vi "Spectrophotometer.vi"() -> ()   [LabVIEW 2015]
uses:
  lamp 3.ctl
  measurement mode.ctl
  standard cluster 2.ctl
  settings.ctl
  sample cluster.ctl
panel:
  in  "Export":bool
  in  "Quick Measure":bool
  in  "Quit":bool
  in  "Mixture Analysis":bool
  in  "Turn Lamp on/off":bool
  in  "Measure reference":bool
  in  "Continuous Sampling":bool
  in  "Print":bool
  in  "Run Pump":bool
  in  "Load Unknowns":bool
  in  "Load Standards":bool
  in  "Measure Unknowns":bool
  in  "Measure Standards":bool
  out "mse":dbl format="%.2e"
  out "Sample cluster":T1={"General description"="", "Sample setup"={"integration time"=0.5, "rinse time"=10.0, "sample time"=10.0, "sample type"=0}, "Absorbance"=[], "Analyst"="", "Sample descriptions"=[], "good data"=[]} {"Absorbance" format="%.2e"; "Sample setup"."sample type" items=["Sample Cuvet", "Sipper Cell", "No Dialog"]; "Sample setup"."sample time" min=0.0 max=100.0 step=1.0 format="%.1f"; "Sample setup"."rinse time" min=0.0 max=100.0 step=1.0 format="%.1f"; "Sample setup"."integration time" format="%.1f"}
  out "standard cluster":T3={"Description"="", "Setup"={"integration time"=0.5, "rinse time"=10.0, "sample time"=10.0, "sample type"=0}, "Concentrations"=[], "Absorbance"=[], "Analyst"="", "Concentration units"="", "Good"=[]} {"Absorbance" format="%.2e"; "Concentrations" format="%.2p"; "Setup"."sample type" items=["Sample Cuvet", "Sipper Cell", "No Dialog"]; "Setup"."sample time" min=0.0 max=100.0 step=1.0 format="%.1f"; "Setup"."rinse time" min=0.0 max=100.0 step=1.0 format="%.1f"; "Setup"."integration time" format="%.1f"}
  out "Max Abs":dbl[](array[numeric])=[2.5701224514044116, 2.7143632947038925, 2.7377490738915573, 2.781755374652469, 2.7830312576242777, 2.8032522114304568, 2.7921527618220714, 2.7673636837963227, 2.7721309273843646, 2.765787727286867, 2.807007059774088, 2.7902851640332416, 2.832726005678466, 2.8510992821765293, 2.8064913329195997, 2.8579954955609237, 2.826035908916132, 2.7882815275987913, 2.827020146123574, 2.862584527170188, 2.8696657972102946, 2.870029150013057, 2.850339854583479, 2.8344461374598717, 2.810178732066239, 2.898747115100364, 2.8854629958743176, 2.8929623242217075, 2.897616096354254, 2.8235133530369914, 2.842072279560508, 2.8740060946591246, 2.8952788625213643, 2.9197995727392203, 2.7718078789991054, 2.7746483290640764, 2.9113813592906737, 2.8881008306142317, 2.8491859254377956, 2.913029295578773, 2.8686091762476096, 2.9204468386734073, 2.88930170250631, 2.884183410137873, 2.874273027848105, 2.8890999188452047, 2.897462138013063, 2.926856708949692, 2.868338737959064, 2.905860615093137, 2.835906080237521, 2.8753391229545393, 2.9027206797044833, 2.7781657266251045, 2.7936088088519138, 2.8090207204836726, 2.809411557915602, 2.8104475951231165, 2.798402011467731, 2.7894114735514233, 2.9238654751855013, 2.9081953926712476, 2.8844894948295754, 2.868914686447694, 2.8460648194194156, 2.933922376656966, 2.9145335490140183, 2.9086029593887113, 2.8939059482930922, 2.893051223353465, 2.884444162559301, 2.889872914270699, 2.885485609489626, 2.896151283804924, 2.8967245808281366, 2.910314846434508, 2.9140468259476626, 2.929408706900379, 2.9352653639533064, 2.9521237832016056, 2.9551680174761126, 2.870181433343178, 2.8722378774668362, 2.8840019247687874, 2.8835592361928204, 2.8905663182570516, 2.8863666233051126, 2.9627101964477114, 2.9386998099696515, 2.91425851170049, 2.9100478084869774, 2.905612412895181, 2.892739996745825, 2.899097900707322, 2.8947147215259488, 2.9053640687668922, 2.9628994480115844, 2.9634572601167077, 2.9468843793177224, 2.964504765269017, 2.9391297105036522, 2.9489506102455483, 2.958143240475256, 2.943237226575327, 2.9568308966253545, 2.957760484109844, 2.925569909543376, 2.9320981608102477, 2.9437318785364797, 2.983147984219146, 2.918565007974718, 2.9265893685399558, 2.940964493492799, 2.9274114291335085, 2.9227877179721355, 2.9445813642269263, 2.9180093558683367, 2.9153470623241917, 2.958516103423041, 2.988112840268352, 2.9362120443202486, 2.988665956710447, 2.915821787620399, 2.9916424442139777, 2.914713286973624, 2.924134497101746, 2.980367026184775, 2.9828770130682005, 2.974695871909683, 2.9668266733534754, 2.9595183769729982, 2.944650435338738, 2.920332071539589, 2.932453470068308, 2.953682391064328, 2.95193947855959, 2.983120894710853, 2.9466487339066765, 2.9510362257417495, 2.970625776688294, 2.962037686565013, 2.963362766103736, 2.9864582127373063, 2.9954070203944414, 2.971758130277843, 2.9846263122003296, 2.9966167306916187, 3.0002344557228784, 2.899535984652174, 2.989627770745151, 2.942959975186675, 2.9796849238270258, 2.9614780469852766, 2.9584683183669434, 2.975275526294007, 2.9971853565284476, 2.992270670437009, 2.9737834204390037, 2.977970397281164, 2.996152530275524, 2.967416919318192, 2.970607188895619, 2.9724250217818824, 2.995977231283496, 2.991305836741952, 2.993991419687998, 2.9771014330008883, 2.989405318001516, 2.9697978489463743, 2.988674872173253, 2.977257059654726, 2.985336641735613, 2.9766800457593336, 2.993241746483962, 2.9943787503552803, 2.9852288183853912, 2.9900367863183996, 2.9793115878060052, 2.993718320050437, 2.9663388811545617, 2.9916158794231995, 2.9982680591088706, 2.9787737843301225, 2.9764416893788446, 2.993938575094718, 2.9830305841443057, 2.9811024954238863, 2.9745853737795214, 2.9796849238270258, 2.9502869470332103, 2.9790837862828363, 2.940556326635444, 3.007577098304339, 2.9971328991685695, 2.9268669879873825, 2.8809621413005586, 2.9915007465494234, 2.986386518883215, 2.893595333819883, 2.8948696567452523, 2.920811805185074, 2.9529860651970554, 2.8761023213777936, 2.9825425823029432, 2.961231197044663, 2.864261824184963, 3.002667047908652, 2.8475849968782785, 2.9785183223473086, 2.966948535845015, 2.976954909894943, 2.9797122285003805, 2.9877466823844996, 2.9517065608430424, 2.973561931079017, 2.9507930951262478, 2.9857945925606715, 2.959251330111692, 2.9697233511042374, 2.9754226169943916, 2.987916403689377, 2.9795847920016643, 2.9802125101844354, 2.9975349104293665, 2.969238803388194, 3.002563443006112, 2.902253164413887, 2.9254668006915376, 2.881567238929719, 2.9765425484286254, 2.982099290774663, 2.9982506175634103, 2.844588996837636, 2.9800306562438332, 2.9985378777712164, 3.0004340774793183, 2.9470610295060045, 2.8992074631292315, 2.8633466564264207, 2.827808515509827, 2.83905045598111, 2.989965680840462, 2.87559367147926, 2.873831919363592, 2.920144205331227, 2.9868165045855366, 2.9401577450345013, 3.0014394694805917, 2.9767167043633824, 3.001949941084268, 2.9683054586308106, 2.995775549929434, 2.988273495044722, 2.9498484576324793, 2.982596831816711, 2.9495461294045358, 2.9017306917292185, 2.9264144800205227, 2.8723544290433782, 2.985857410884626, 2.941163460158473, 2.938989289805111, 2.981066205174902, 2.990817735602789, 2.8994374542861774, 2.9779064276371185, 2.9417796781737486, 2.9370964319634765, 2.981963498779465, 3.0066286048286996, 2.9856150615513544, 3.0025202670010356, 2.9894854141161935, 2.9764141782996054, 2.978271841610635, 3.004699604225055, 2.984787811891183, 2.963277703909644, 2.9347407805432075, 2.985480364573659, 2.9774400784660493, 2.983193129645013, 2.9729795213258945, 2.9958106316760427, 2.9554087118535692, 2.9892183696006756, 2.9759829437125465, 2.9923060364371836, 2.9796212062457554, 2.9712846644554203, 2.9653334280184214, 2.968277427274059, 2.9958194016699227, 2.928825836692016, 2.913866811896239, 2.9962401532444884, 2.989075878689533, 3.002407989295258, 2.958085848521085, 2.9812381033887854, 3.0012922730241685, 2.9299703849090117, 2.972072715743075, 3.010850957373923, 2.865743391885155, 2.895024536710891, 2.8531260748344462, 2.8453461374114086, 2.8730996193611147, 2.976056375590289, 2.8718997009048017, 2.809855876532671, 2.7851019486186024, 2.8378030074943434, 2.751048034820188, 2.7677938472611476] format="%.2f"
  out "Sample absorbance":dbl[](array[numeric])=[0.07717] format="%.4f"
  out "concentration":dbl=0.0001 format="%.1e"
  in  "measurement mode":T4 {"gain" max=15}
  out "lamp":T5
  out "max. conc.":dbl format="%.2p"
  out "reference":bool=TRUE
  out "calibration graph":cluster{dbl[], dbl[]}[](graph)
  out "Sample concentration":dbl[](array[numeric])=[0.00011953621702929448] format="%.2e"
  out "Sample description":string[](array[string])
  out "Samples graph":cluster{sgl, sgl, dbl[][]}(graph)
  out "r":dbl format="%.4f"
  out "intercept":dbl format="%.2e"
  out "slope":dbl format="%.3e"
  in  "GPIB":string="18"
  out "Standards graph":cluster{sgl, sgl, dbl[][]}(graph)
  # "nm"
  # "absorbance"
  # "Calibration graph"
  # "Description"
  # "Absorbance"
  # "Concentration"
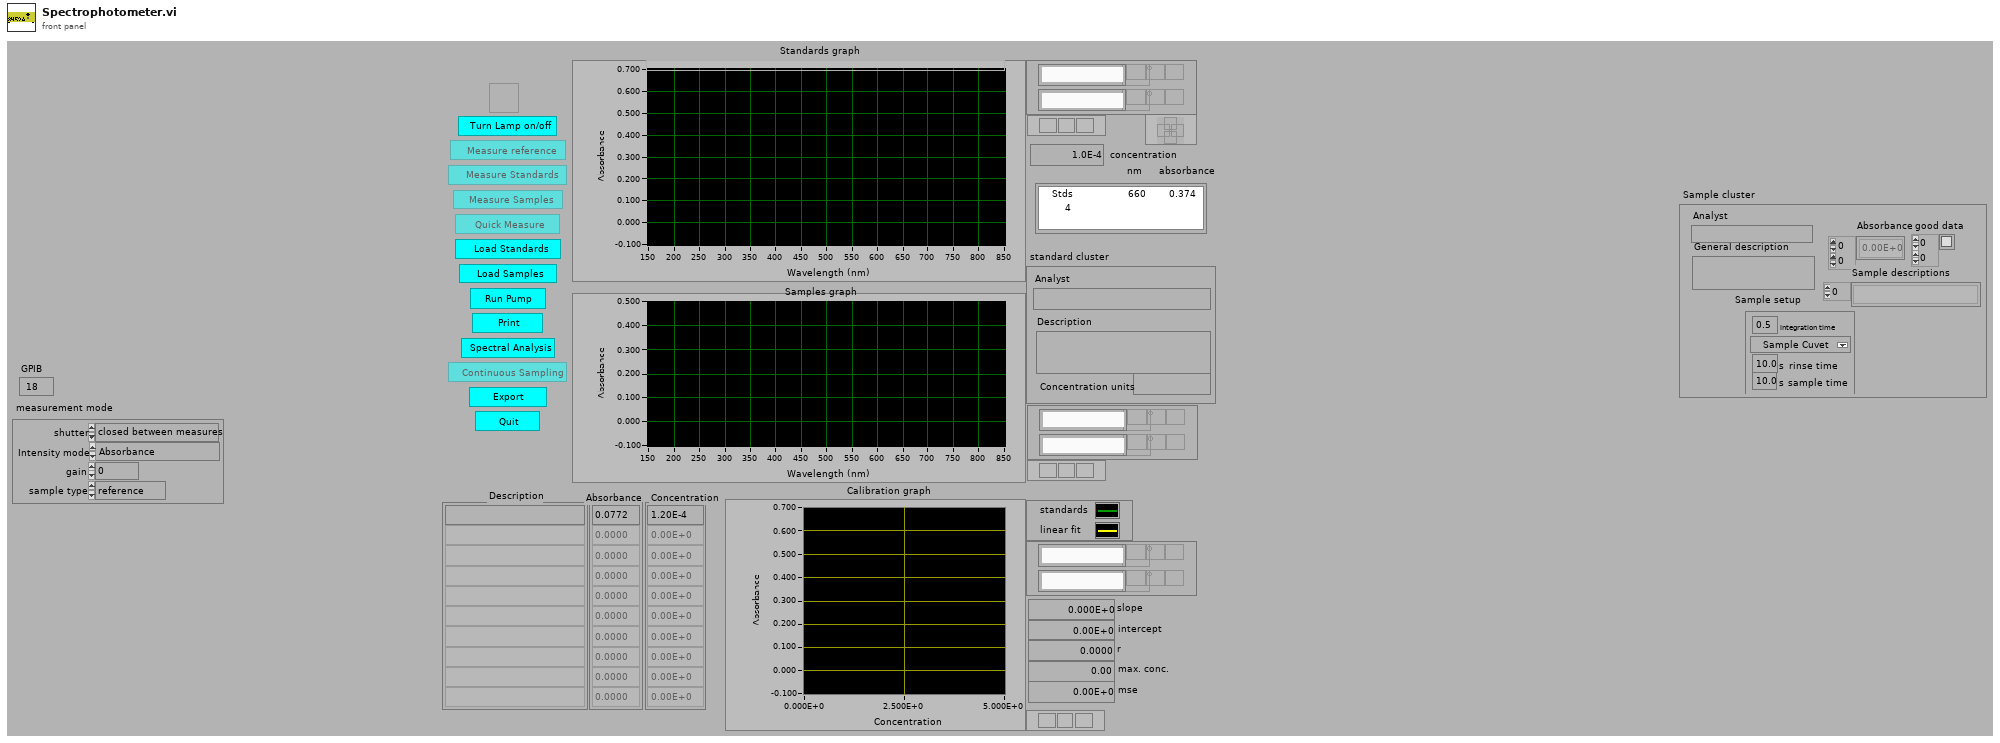
[diagram p1: front panel]
types:
  T1 = typedef "sample cluster.ctl" = cluster{"General description":string, "Sample setup":T2, "Absorbance":dbl[][], "Analyst":string, "Sample descriptions":string[], "good data":bool[][]}
  T2 = typedef "settings.ctl" = cluster{"integration time":sgl, "rinse time":dbl[unit], "sample time":dbl[unit], "sample type":u16}
  T3 = typedef "standard cluster 2.ctl" = cluster{"Description":string, "Setup":T2, "Concentrations":dbl[], "Absorbance":dbl[][], "Analyst":string, "Concentration units":string, "Good":bool[][]}
  T4 = typedef "measurement mode.ctl" = cluster{"shutter":enum16{"closed between measures", "open between measures"}, "Intensity mode":enum16{"Absorbance", "Intensity at current gain", "Intensity at fixed gain", "dark current at current gain", "dark current at fixed gain"}, "gain":u8, "sample type":enum16{"reference", "standard", "unknown", "Diagnostic"}}
  T5 = typedef "lamp 3.ctl" = bool
  T6 = enum16{"reference", "standard", "unknown", "Diagnostic"}
  T7 = typedef "lamp2.ctl" = bool
  T8 = typedef "standard cluster.ctl" = cluster{"Description":string, "Setup":T2, "Concentrations":dbl[], "Absorbance":dbl[][], "Analyst":string, "Concentration units":string, "Good":bool[][]}
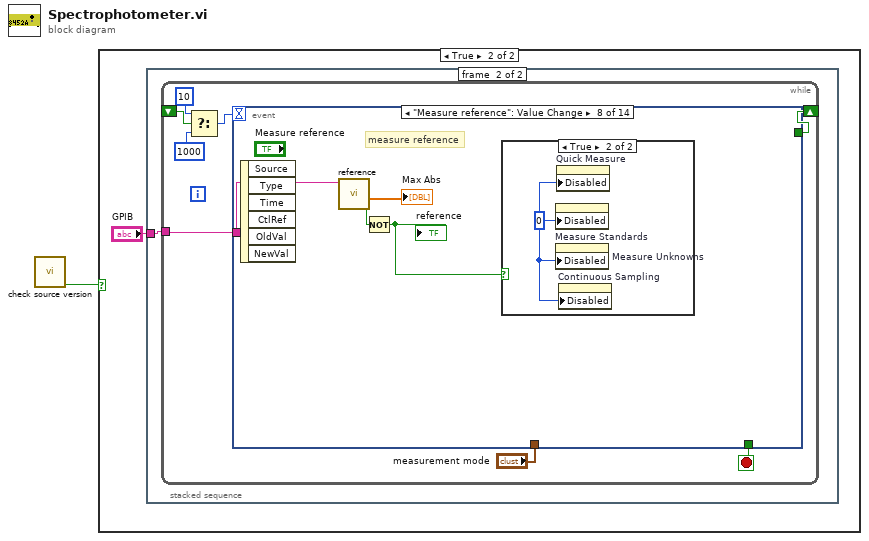
[diagram p0: block diagram]
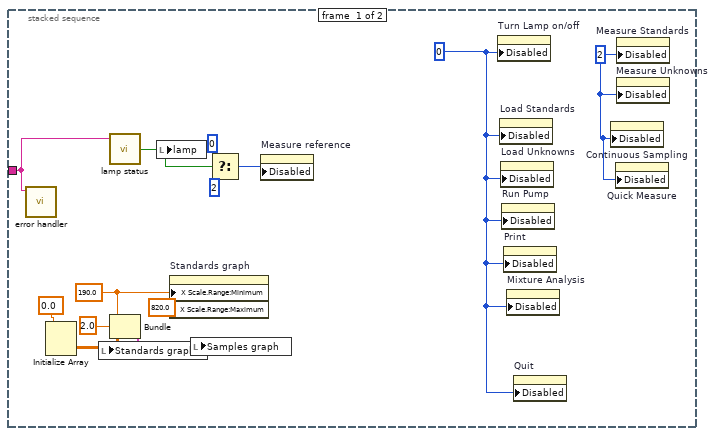
[diagram p3: hidden frame]
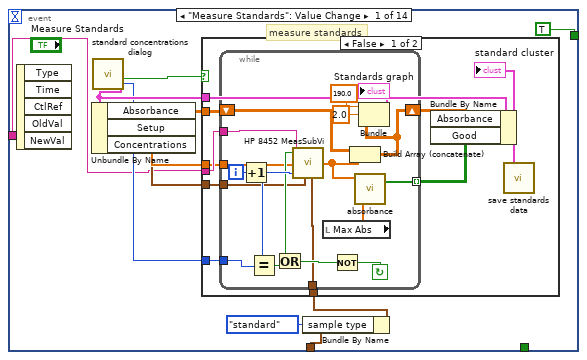
[diagram p4: hidden frame]
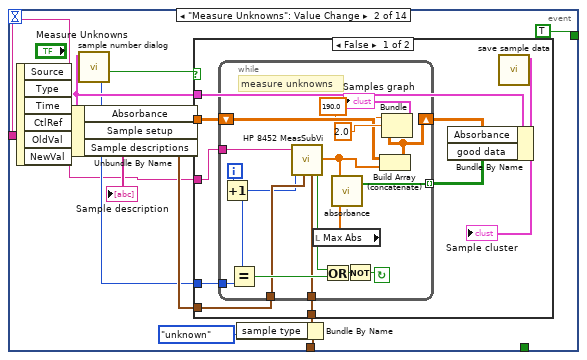
[diagram p6: hidden frame]
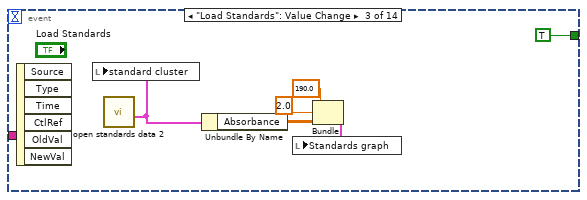
[diagram p8: hidden frame]
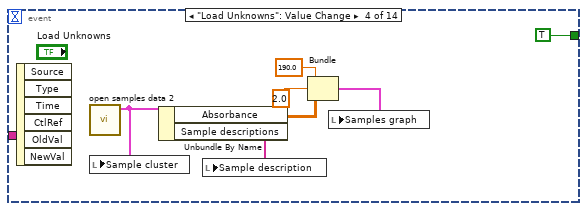
[diagram p9: hidden frame]
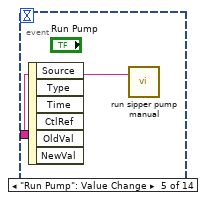
[diagram p10: hidden frame]
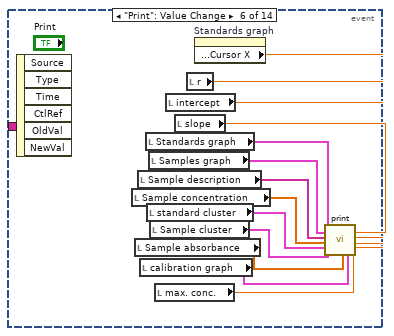
[diagram p11: hidden frame]
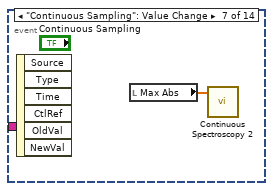
[diagram p12: hidden frame]
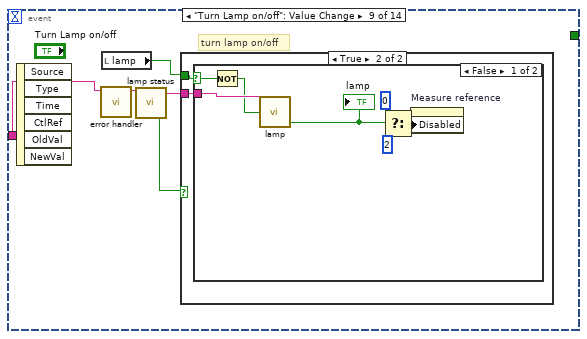
[diagram p14: hidden frame]
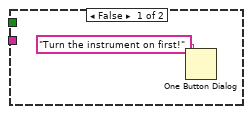
[diagram p15: hidden frame]
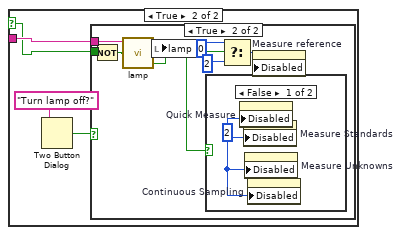
[diagram p16: hidden frame]
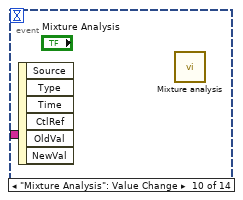
[diagram p19: hidden frame]
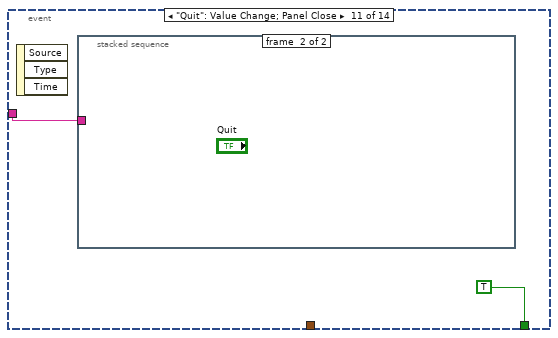
[diagram p20: hidden frame]
diagram:
  n1 = call "check source version.vi"() -> ("continue running?"=w1:bool)  [unwired: 2 in, 3 out]
  n2 = case shown="True" w1 {
    frame False {
    }
    frame True {
      n3 = stacked-sequence {
        tunnel: "GPIB" -> [w10 w16]
        frame #0 {
          w3 = 2
          w11 = 0
          w13 = sgl 190.0
          n4 = call "error handler.vi"("GPIB in"=w10) -> ()  [unwired: 4 in, 3 out]
          n5 = Initialize Array(0.0) -> (w5:dbl[][])  [unwired: 2 in]
          n6 = call "lamp status.vi"("GPIB in"=w10) -> ("lamp"=w6:T7)  [unwired: 2 in, 2 out]
          n7 = Bundle(w13, sgl 2.0, w5) -> (w4:cluster{sgl, sgl, dbl[][]})  [unwired: 1 in]
          n8 = local write "Standards graph"(w4) -> ()
          n9 = local write "lamp"(w6) -> ()
          n10 = property on="Standards graph" class="WFGraph (strict)"("X Scale.Range:Minimum"=w13, "X Scale.Range:Maximum"=sgl 820.0) -> ()  [unwired: 2 in, 2 out]
          n11 = local write "Samples graph"(w4) -> ()
          n12 = Select(t=0, s=w6, f=2) -> (s? t:f=w7:i32)
          n13 = property on="Measure reference" class="Bool"("Disabled"=w7) -> ()  [unwired: 2 in, 2 out]
          n14 = property on="Turn Lamp on/off" class="Bool"("Disabled"=w11) -> ()  [unwired: 2 in, 2 out]
          n15 = property on="Load Standards" class="Bool"("Disabled"=w11) -> ()  [unwired: 2 in, 2 out]
          n16 = property on="Load Unknowns" class="Bool"("Disabled"=w11) -> ()  [unwired: 2 in, 2 out]
          n17 = property on="Run Pump" class="Bool"("Disabled"=w11) -> ()  [unwired: 2 in, 2 out]
          n18 = property on="Print" class="Bool"("Disabled"=w11) -> ()  [unwired: 2 in, 2 out]
          n19 = property on="Mixture Analysis" class="Bool"("Disabled"=w11) -> ()  [unwired: 2 in, 2 out]
          n20 = property on="Quit" class="Bool"("Disabled"=w11) -> ()  [unwired: 2 in, 2 out]
          n21 = property on="Continuous Sampling" class="Bool"("Disabled"=w3) -> ()  [unwired: 2 in, 2 out]
          n22 = property on="Quick Measure" class="Bool"("Disabled"=w3) -> ()  [unwired: 2 in, 2 out]
          n23 = property on="Measure Standards" class="Bool"("Disabled"=w3) -> ()  [unwired: 2 in, 2 out]
          n24 = property on="Measure Unknowns" class="Bool"("Disabled"=w3) -> ()  [unwired: 2 in, 2 out]
        }
        frame #1 {
          n25 = while {
            tunnel: w16 -> [w22]
            shift-right: [w19] -> _
            shift-left: _ -> [w18]
            stop <- w23 stop-if-true
            n26 = Select(t=10, s=w18, f=1000) -> (s? t:f=w17:i32)
            n27 = event shown="[7] \"Measure reference\": Value Change" {
              selector: _ -> [_ _ _ _ _ _ _ _ _ _ _ _ _ _]
              dyn-events: _ -> [_ _ _ _ _ _ _ _ _ _ _ _ _ _]
              timeout: w17 -> [_ _ _ _ _ _ _ _ _ _ _ _ _ _]
              tunnel: w22 -> [w28 w67 _ _ w116 _ _ w131 w136 _ w164 w176 w199 _]
              tunnel: "measurement mode" -> [w27 w68 _ _ _ _ _ _ _ _ _ _ w198 _]
              tunnel: [_ _ _ _ _ _ _ _ _ _ TRUE ("Quit") _ _ _] -> w23
              tunnel: [TRUE TRUE TRUE TRUE _ _ _ _ _ _ _ FALSE TRUE _] -> w19
              event "Measure Standards": Value Change {
                n28 = event-data() -> ()  [unwired: 1 in, 5 out]
                n29 = call "standard concentrations dialog"() -> ("canceled"=w31:bool, "number"=w29:i8, "standard cluster"=w34:T8)  [unwired: 9 in]
                n30 = Unbundle By Name(w34) -> ("Absorbance"=w33:dbl[][], "Setup"=w32:T2, "Concentrations"=w35:dbl[])
                n31 = Bundle By Name(cluster=w27, "sample type"=T6."standard") -> (w30:T4)
                n32 = case shown="False" w31 {
                  tunnel: w28 -> [w45 _]
                  tunnel: w30 -> [w44 _]
                  tunnel: w29 -> [w43 _]
                  tunnel: w33 -> [w42 _]
                  tunnel: w32 -> [w41 _]
                  tunnel: w34 -> [w40 _]
                  tunnel: w35 -> [w37 _]
                  frame False {
                    # "measure standards"
                    n33 = while {
                      tunnel: w37 -> [w47]
                      tunnel: [w48] -> w38 mode=indexing
                      tunnel: w41 -> [w50]
                      tunnel: w44 -> [w52]
                      tunnel: w43 -> [w56]
                      tunnel: w45 -> [w55]
                      shift-left: w42 -> [w64]
                      shift-right: [w63] -> w39
                      i -> [w61]
                      stop <- w57 continue-if-true
                      n34 = Increment(x=w61) -> (x+1=w54:i32)
                      n35 = Equal?(x=w54, y=w56) -> (x = y?=w59:bool)
                      n36 = call "HP 8452 MeasSubVi.vi"("GPIB in"=w55, "Standard"=w47, "sample number"=w54, "setup"=w50, "measurement mode"=w52) -> ("canceled"=w53:bool, "measurement"=w49:dbl[])  [unwired: 2 in, 1 out]
                      n37 = Or(x=w53, y=w59) -> (x .or. y?=w58:bool)
                      n38 = local read "Max Abs"() -> (w51:dbl[])
                      n39 = Not(x=w58) -> (.not. x?=w57:bool)
                      n40 = Build Array (concatenate)(w64, w49) -> (w63:dbl[][])
                      n41 = call "absorbance.vi"("Amax"=w51, "Asample"=w49) -> ("good data"=w48:bool[])  [unwired: 3 in]
                      n42 = Bundle(sgl 190.0, sgl 2.0, w63) -> (→"Standards graph":cluster{sgl, sgl, dbl[][]})  [unwired: 1 in]
                    }
                    n43 = Bundle By Name(cluster=w40, "Absorbance"=w39, "Good"=w38) -> (w36:T8)
                    "standard cluster" <- w36
                    n44 = call "save standards data.vi"("standard cluster"=w36) -> ()  [unwired: 5 in]
                  }
                  frame True {
                  }
                }
              }
              event "Measure Unknowns": Value Change {
                n45 = event-data() -> ()  [unwired: 1 in, 6 out]
                n46 = call "sample number dialog"() -> ("canceled"=w71:bool, "number"=w69:i8, "Sample cluster"=w75:T1)  [unwired: 9 in]
                n47 = Unbundle By Name(w75) -> ("Absorbance"=w72:dbl[][], "Sample setup"=w73:T2, "Sample descriptions"=→"Sample description":string[])
                n48 = Bundle By Name(cluster=w68, "sample type"=T6."unknown") -> (w70:T4)
                n49 = case shown="False" w71 {
                  tunnel: w73 -> [w81 _]
                  tunnel: w67 -> [w84 _]
                  tunnel: w70 -> [w83 _]
                  tunnel: w69 -> [w82 _]
                  tunnel: w72 -> [w80 _]
                  tunnel: w75 -> [w79 _]
                  frame False {
                    n50 = while {
                      tunnel: [w86] -> w77 mode=indexing
                      tunnel: w83 -> [w92]
                      tunnel: w82 -> [w99]
                      tunnel: w81 -> [w93]
                      tunnel: w84 -> [w91]
                      shift-left: w80 -> [w89]
                      shift-right: [w102] -> w76
                      i -> [w98]
                      stop <- w95 continue-if-true
                      # "measure unknowns"
                      n51 = Increment(x=w98) -> (x+1=w90:i32)
                      n52 = Equal?(x=w90, y=w99) -> (x = y?=w97:bool)
                      n53 = call "HP 8452 MeasSubVi.vi"("GPIB in"=w91, "sample number"=w90, "setup"=w93, "measurement mode"=w92) -> ("canceled"=w94:bool, "measurement"=w87:dbl[])  [unwired: 3 in, 1 out]
                      n54 = local read "Max Abs"() -> (w88:dbl[])
                      n55 = Or(x=w94, y=w97) -> (x .or. y?=w96:bool)
                      n56 = call "absorbance.vi"("Amax"=w88, "Asample"=w87) -> ("good data"=w86:bool[])  [unwired: 3 in]
                      n57 = Not(x=w96) -> (.not. x?=w95:bool)
                      n58 = Build Array (concatenate)(w89, w87) -> (w102:dbl[][])
                      n59 = Bundle(sgl 190.0, sgl 2.0, w102) -> (→"Samples graph":cluster{sgl, sgl, dbl[][]})  [unwired: 1 in]
                    }
                    n60 = Bundle By Name(cluster=w79, "Absorbance"=w76, "good data"=w77) -> (w78:T1)
                    "Sample cluster" <- w78
                    n61 = call "save sample data.vi"("Sample cluster"=w78) -> ()  [unwired: 5 in]
                  }
                  frame True {
                  }
                }
              }
              event "Load Standards": Value Change {
                n62 = event-data() -> ()  [unwired: 1 in, 6 out]
                n63 = call "open standards data 2.vi"() -> ("standard cluster"=w105:T8)  [unwired: 9 in, 2 out]
                n64 = local write "standard cluster"(w105) -> ()
                n65 = Unbundle By Name(w105) -> ("Absorbance"=w106:dbl[][])
                n66 = Bundle(sgl 190.0, sgl 2.0, "Absorbance"=w106) -> (w107:cluster{sgl, sgl, "Absorbance":dbl[][]})  [unwired: 1 in]
                n67 = local write "Standards graph"(w107) -> ()
              }
              event "Load Unknowns": Value Change {
                n68 = event-data() -> ()  [unwired: 1 in, 6 out]
                n69 = call "open samples data 2.vi"() -> ("Sample cluster"=w113:T1)  [unwired: 7 in]
                n70 = local write "Sample cluster"(w113) -> ()
                n71 = Unbundle By Name(w113) -> ("Absorbance"=w112:dbl[][], "Sample descriptions"=w115:string[])
                n72 = local write "Sample description"(w115) -> ()
                n73 = Bundle(sgl 190.0, sgl 2.0, "Absorbance"=w112) -> (w111:cluster{sgl, sgl, "Absorbance":dbl[][]})  [unwired: 1 in]
                n74 = local write "Samples graph"(w111) -> ()
              }
              event "Run Pump": Value Change {
                n75 = event-data() -> ()  [unwired: 1 in, 6 out]
                n76 = call "run sipper pump manual.vi"("GPIB in"=w116) -> ()  [unwired: 3 in]
              }
              event "Print": Value Change {
                n77 = event-data() -> ()  [unwired: 1 in, 6 out]
                n78 = local read "Sample concentration"() -> (w123:dbl[])
                n79 = local read "Sample absorbance"() -> (w126:dbl[])
                n80 = local read "Sample description"() -> (w122:string[])
                n81 = local read "calibration graph"() -> (w127:cluster{dbl[], dbl[]}[])
                n82 = local read "Standards graph"() -> (w120:cluster{sgl, sgl, dbl[][]})
                n83 = local read "standard cluster"() -> (w124:T3)
                n84 = local read "Samples graph"() -> (w121:cluster{sgl, sgl, dbl[][]})
                n85 = local read "Sample cluster"() -> (w125:T1)
                n86 = local read "max. conc."() -> (w128:dbl)
                n87 = local read "intercept"() -> (w118:dbl)
                n88 = local read "slope"() -> (w119:dbl)
                n89 = local read "r"() -> (w117:dbl)
                n90 = property on="Standards graph" class="WFGraph (strict)"() -> ("Cursor.Cursor Position:Cursor X"=w129:dbl)  [unwired: 2 in, 2 out]
                n91 = call "print.vi"("Standard graph"=w120, "Unknowns graph"=w121, "Sample description"=w122, "Sample  concentration"=w123, "standard cluster"=w124, "Sample cluster"=w125, "Unknown absorbance"=w126, "calibration graph"=w127, "slope"=w119, "intercept"=w118, "r"=w117, "wavelength"=w129, "max. conc."=w128) -> ()  [unwired: 7 in]
              }
              event "Continuous Sampling": Value Change {
                n92 = event-data() -> ()  [unwired: 1 in, 6 out]
                n93 = local read "Max Abs"() -> (w130:dbl[])
                n94 = call "Continuous Spectroscopy 2"("Max Abs"=w130) -> ()  [unwired: 11 in]
              }
              event "Measure reference": Value Change {
                # "measure reference"
                n95 = event-data() -> ()  [unwired: 1 in, 6 out]
                n96 = call "reference.vi"("GPIB"=w131) -> ("canceled"=w133:bool, "Amax"=→"Max Abs":dbl[])  [unwired: 6 in, 2 out]
                n97 = Not(x=w133) -> (.not. x?=w134:bool)
                "reference" <- w134
                n98 = case shown="True" w134 {
                  frame False {
                  }
                  frame True {
                    w135 = 0
                    n99 = property on="Measure Standards" class="Bool"("Disabled"=w135) -> ()  [unwired: 2 in, 2 out]
                    n100 = property on="Measure Unknowns" class="Bool"("Disabled"=w135) -> ()  [unwired: 2 in, 2 out]
                    n101 = property on="Quick Measure" class="Bool"("Disabled"=w135) -> ()  [unwired: 2 in, 2 out]
                    n102 = property on="Continuous Sampling" class="Bool"("Disabled"=w135) -> ()  [unwired: 2 in, 2 out]
                  }
                }
              }
              event "Turn Lamp on/off": Value Change {
                # "turn lamp on/off"
                n103 = event-data() -> ()  [unwired: 1 in, 6 out]
                n104 = call "error handler.vi"("GPIB in"=w136) -> ("GPIB out"=w137:string)  [unwired: 4 in, 2 out]
                n105 = local read "lamp"() -> (w140:T5)
                n106 = call "lamp status.vi"("GPIB in"=w137) -> ("instrument on"=w139:bool, "GPIB out"=w138:string)  [unwired: 2 in, 1 out]
                n107 = case shown="True" w139 {
                  tunnel: w138 -> [_ w143]
                  tunnel: w140 -> [_ w142]
                  frame False {
                    n108 = One Button Dialog(message="Turn the instrument on first!") -> ()  [unwired: 1 in, 1 out]
                  }
                  frame True {
                    n109 = case shown="False" w142 {
                      selector: w142 -> [w145 w151]
                      tunnel: w143 -> [w150 w152]
                      frame False {
                        n110 = Not(x=w145) -> (.not. x?=w144:bool)
                        n111 = call "lamp.vi"("lamp"=w144, "GPIB in"=w150) -> ("lamp okay"=w146:bool)  [unwired: 2 in, 1 out]
                        "lamp" <- w146
                        n112 = Select(t=0, s=w146, f=2) -> (s? t:f=w149:i32)
                        n113 = property on="Measure reference" class="Bool"("Disabled"=w149) -> ()  [unwired: 2 in, 2 out]
                      }
                      frame True {
                        n114 = Two Button Dialog(message="Turn lamp off?") -> (T button?=w153:bool)  [unwired: 2 in]
                        n115 = case shown="True" w153 {
                          tunnel: w151 -> [_ w158]
                          tunnel: w152 -> [_ w157]
                          frame False {
                          }
                          frame True {
                            n116 = Not(x=w158) -> (.not. x?=w156:bool)
                            n117 = call "lamp.vi"("lamp"=w156, "GPIB in"=w157) -> ("lamp okay"=w155:bool)  [unwired: 2 in, 1 out]
                            n118 = local write "lamp"(w155) -> ()
                            n119 = case shown="False" w155 {
                              frame False {
                                w162 = 2
                                n120 = property on="Quick Measure" class="Bool"("Disabled"=w162) -> ()  [unwired: 2 in, 2 out]
                                n121 = property on="Measure Standards" class="Bool"("Disabled"=w162) -> ()  [unwired: 2 in, 2 out]
                                n122 = property on="Measure Unknowns" class="Bool"("Disabled"=w162) -> ()  [unwired: 2 in, 2 out]
                                n123 = property on="Continuous Sampling" class="Bool"("Disabled"=w162) -> ()  [unwired: 2 in, 2 out]
                              }
                              frame True {
                              }
                            }
                            n124 = Select(t=0, s=w155, f=2) -> (s? t:f=w159:i32)
                            n125 = property on="Measure reference" class="Bool"("Disabled"=w159) -> ()  [unwired: 2 in, 2 out]
                          }
                        }
                      }
                    }
                  }
                }
              }
              event "Mixture Analysis": Value Change {
                n126 = event-data() -> ()  [unwired: 1 in, 6 out]
                n127 = call "Mixture analysis"() -> ()  [unwired: 1 in]
              }
              event "Quit": Value Change; Panel Close {
                n128 = event-data() -> ()  [unwired: 1 in, 3 out]
                n129 = stacked-sequence {
                  tunnel: w164 -> [w165 _]
                  frame #0 {
                    n130 = local read "lamp"() -> (w166:T5)
                    n131 = case shown="True" w166 {
                      tunnel: w165 -> [_ w171]
                      frame False {
                      }
                      frame True {
                        n132 = Two Button Dialog(message="Do you want to turn off the lamp", 1:"No", 2:"Yes") -> (T button?=w170:bool)
                        n133 = case shown="True" w170 {
                          tunnel: w171 -> [_ w173]
                          frame False {
                          }
                          frame True {
                            n134 = call "lamp.vi"("lamp"=FALSE, "GPIB in"=w173) -> ()  [unwired: 2 in, 2 out]
                          }
                        }
                      }
                    }
                  }
                  frame #1 {
                  }
                }
              }
              event "Standards graph": Mouse Up; Timeout {
                # "estimate unknowns"
                n135 = event-data() -> ()  [unwired: 1 in, 3 out]
                n136 = local read "standard cluster"() -> (w191:T3)
                n137 = call "lamp status.vi"("GPIB in"=w176) -> ("lamp"=w180:T7)  [unwired: 2 in, 2 out]
                n138 = local read "Sample cluster"() -> (w192:T1)
                n139 = Unbundle By Name(w191) -> ("Concentrations"=w181:dbl[])
                n140 = property on="Standards graph" class="WFGraph (strict)"() -> ("Cursor.Cursor Position:Cursor X"=w174:dbl)  [unwired: 2 in, 2 out]
                n141 = local write "lamp"(w180) -> ()
                n142 = Select(t=0, s=w180, f=2) -> (s? t:f=w177:i32)
                n143 = property on="Measure reference" class="Bool"("Disabled"=w177) -> ()  [unwired: 2 in, 2 out]
                n144 = call "calculate unknowns"("Calibration wavelength"=w174, "Sample cluster"=w192, "standard cluster"=w191) -> ("Sample  absorbance"=→"Sample absorbance":dbl[], "slope"=→"slope":dbl, "intercept"=→"intercept":dbl, "r"=→"r":dbl, "Sample  concentration"=→"Sample concentration":dbl[], "mse"=→"mse":dbl, "Max. Conc."=→"max. conc.":dbl, "graph"=→"calibration graph":cluster{dbl[], dbl[]}[])  [unwired: 5 in]
                n145 = case shown="False" w180 {
                  frame False {
                    w195 = 2
                    n146 = property on="Measure Standards" class="Bool"("Disabled"=w195) -> ()  [unwired: 2 in, 2 out]
                    n147 = property on="Measure Unknowns" class="Bool"("Disabled"=w195) -> ()  [unwired: 2 in, 2 out]
                    n148 = property on="Continuous Sampling" class="Bool"("Disabled"=w195) -> ()  [unwired: 2 in, 2 out]
                  }
                  frame True {
                  }
                }
                n149 = property on="Standards graph" class="WFGraph (strict)"() -> ("Cursor.Cursor Position:Cursor X"=w190:dbl, "Cursor.Cursor Plot"=w188:i32)  [unwired: 2 in, 2 out]
                n150 = Index Array(array=w181, index=w188) -> (element=→"concentration":dbl)
                n151 = property on="Samples graph" class="WFGraph (strict)"("Cursor.Cursor Position:Cursor X"=w190) -> ()  [unwired: 2 in, 2 out]
              }
              event "Quick Measure": Value Change {
                w209 = dbl[unit] 0.0  # s
                w208 = dbl[unit] 0.0  # s
                n152 = event-data() -> ()  [unwired: 1 in, 6 out]
                n153 = Bundle(0.5, w208, w209, i8 2) -> (w215:cluster{dbl, dbl[unit], dbl[unit], i8})  [unwired: 1 in]
                n154 = Bundle By Name(cluster=w198, "sample type"=T6."unknown") -> (w200:T4)
                n155 = call "HP 8452 MeasSubVi.vi"("GPIB in"=w199, "sample number"=1, "setup"=w215, "measurement mode"=w200) -> ("measurement"=w202:dbl[])  [unwired: 3 in, 2 out]
                n156 = local read "Max Abs"() -> (w203:dbl[])
                n157 = call "absorbance.vi"("Amax"=w203, "Asample"=w202) -> ("good data"=w210:bool[])  [unwired: 3 in]
                n158 = Build Array(w210) -> (w213:bool[][])
                n159 = Build Array(w202) -> (w214:dbl[][])
                n160 = Bundle(sgl 190.0, sgl 2.0, w214) -> (w206:cluster{sgl, sgl, dbl[][]})  [unwired: 1 in]
                n161 = local write "Samples graph"(w206) -> ()
                n162 = local read "Sample cluster"() -> (w211:T1)
                n163 = Bundle By Name(cluster=w211, "Sample setup"=w215, "Absorbance"=w214, "good data"=w213) -> (w212:T1)
                n164 = local write "Sample cluster"(w212) -> ()
              }
              event "Export": Value Change {
                n165 = event-data() -> ()  [unwired: 1 in, 6 out]
                n166 = local read "standard cluster"() -> (w217:T3)
                n167 = local read "Sample cluster"() -> (w218:T1)
                n168 = call "export spectra.vi"("Sample cluster"=w218, "standard cluster"=w217) -> ()  [unwired: 10 in]
              }
            }
          }
        }
      }
    }
  }
